vi "destroyEventActuatorTestStatus.vi"(8 "error in (no error)":errorcluster, 11 "UserEvents in":refnum<class "UserEvents.lvclass">) -> (0 "error out":errorcluster, 3 "UserEvents out":refnum<class "UserEvents.lvclass">)   [LabVIEW 2016, in "UserEvents.lvclass"]
uses:
  UserEvents.lvclass
  UserEvents.lvclass/UserEvents.ctl
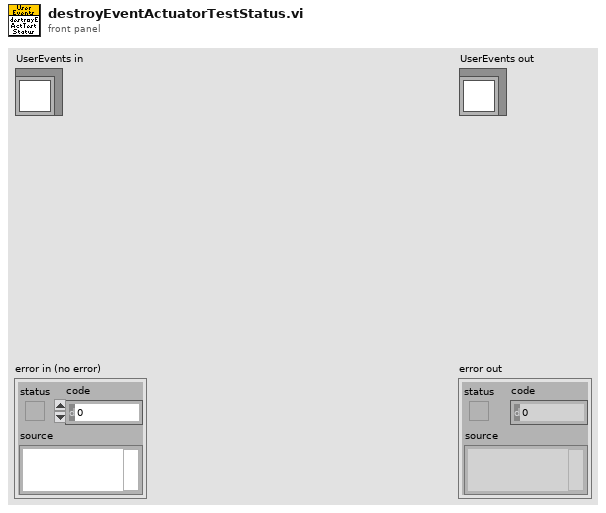
[diagram p1: front panel]
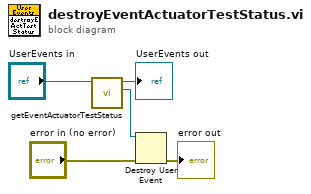
[diagram p0: block diagram]
diagram:
  n1 = call "getEventActuatorTestStatus.vi"("UserEvents in"="UserEvents in") -> ("EventActuatorTestStatus"=w1:refnum<user-event>, "UserEvents out"=→"UserEvents out":refnum<class "UserEvents.lvclass">)  [unwired: 9 in]
  n2 = Destroy User Event(user event=w1, error in="error in (no error)") -> (error out=→"error out":errorcluster)
